vi "ClimbTeleop.vi"(10 "Down?":bool, 11 "Up?":bool) -> ()   [LabVIEW 2018]
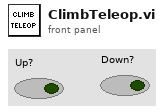
[diagram p1: front panel]
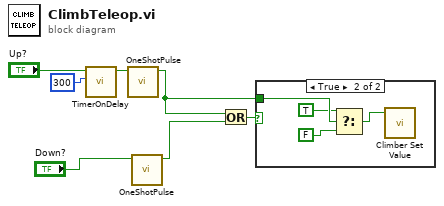
[diagram p0: block diagram]
diagram:
  n1 = call "TimerOnDelay.vi"("Time Limit"=u32 300, "Input"="Up?") -> ("Output"=w1:bool)  [unwired: 9 in]
  n2 = call "OneShotPulse.vi"("Input"=w1) -> ("Output"=w4:bool)  [unwired: 10 in]
  n3 = call "OneShotPulse.vi"("Input"="Down?") -> ("Output"=w5:bool)  [unwired: 10 in]
  n4 = Or(x=w4, y=w5) -> (x .or. y?=w7:bool)
  n5 = case shown="True" w7 {
    tunnel: w4 -> [_ w11]
    frame False {
    }
    frame True {
      n6 = Select(t=TRUE, s=w11, f=FALSE) -> (s? t:f=w8:bool)
      n7 = call "Climber Set Value.vi"("Up?"=w8) -> ()  [unwired: 10 in, 1 out]
    }
  }
